vi "LinearSystemLoop_ClampInput.vi"(9 "UnclampedU":T1, 11 "input inear System Loop":T2) -> (3 "U":T1)   [LabVIEW 2019, in "Trajectory_Library.lvlib"]
doc: "Creates a new LINEAR SYSTEM data cluster with the specified values. \n\n\nInputs: \n - XXX -- XXX.\n\nOutputs:\n - XXX -- XXX."
uses:
  Trajectory_Library.lvlib
  <vilib>/Analysis/Matrix/Datatypes/RealMatrix.ctl
  LINEAR_SYSTEM_LOOP.ctl
  LINEAR_QUADRATIC_REGULATOR.ctl
  LINEAR_PLANT_INV_FF.ctl
  KALMAN_FILTER.ctl
  LINEAR_SYSTEM.ctl
  <vilib>/Analysis/Matrix/NI_Matrix.lvlib
panel:
  # "<States,1>"
  # "<FUTURE --- CLAMP TYPE -- For now\nuse Normalize>"
  # "Steady State Gain  \n<States,Outputs>"
  # "State Estimate <Statess,1>"
  # "<States,States>"
  # "<States,Inputs>"
  # "<Outputs,States>"
  # "<Outputs,Inputs>"
  # "<States,1>"
  # "<Inputs,1>"
  # "<States,Inputs>"
  # "<States,States>"
  # "Ref State <States,1>"
  # "Comp and capped \noutput <Inputs,1>"
  # "Controller gain\n<Inputs,States>"
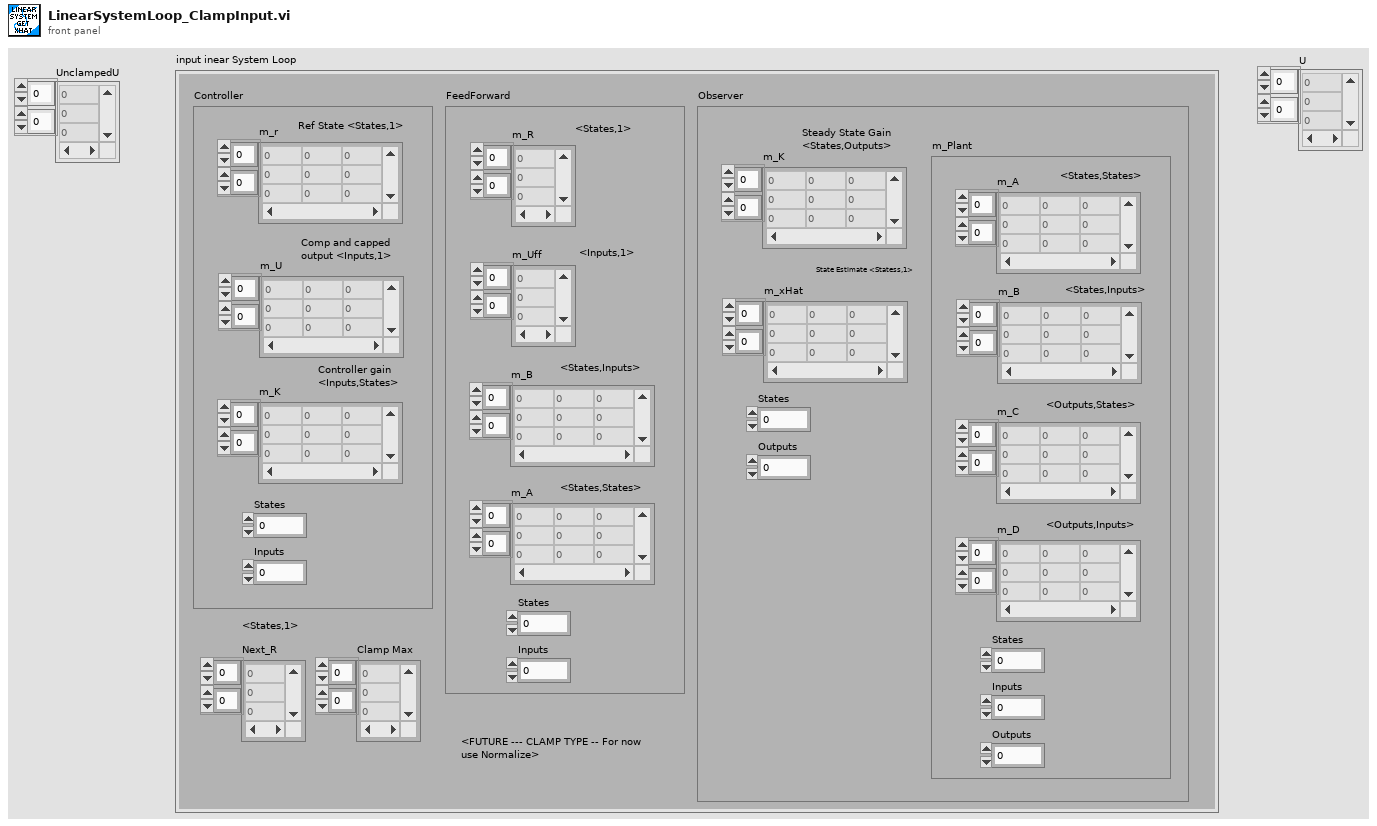
[diagram p1: front panel]
types:
  T1 = typedef "NI_Matrix.lvlib/RealMatrix.ctl" = dbl[][]
  T2 = typedef "Trajectory_Library.lvlib/LINEAR_SYSTEM_LOOP.ctl" = cluster{"Controller":T3, "FeedForward":T4, "Observer":T5, "Next_R":T1, "Clamp Max":T1}
  T3 = typedef "Trajectory_Library.lvlib/LINEAR_QUADRATIC_REGULATOR.ctl" = cluster{"m_r":T1, "m_U":T1, "m_K":T1, "States":i32, "Inputs":i32}
  T4 = typedef "Trajectory_Library.lvlib/LINEAR_PLANT_INV_FF.ctl" = cluster{"m_R":T1, "m_Uff":T1, "m_B":T1, "m_A":T1, "States":i32, "Inputs":i32}
  T5 = typedef "Trajectory_Library.lvlib/KALMAN_FILTER.ctl" = cluster{"m_K":T1, "m_xHat":T1, "States":i32, "Outputs":i32, "m_Plant":T6}
  T6 = typedef "Trajectory_Library.lvlib/LINEAR_SYSTEM.ctl" = cluster{"m_A":T1, "m_B":T1, "m_C":T1, "m_D":T1, "States":i32, "Inputs":i32, "Outputs":i32}
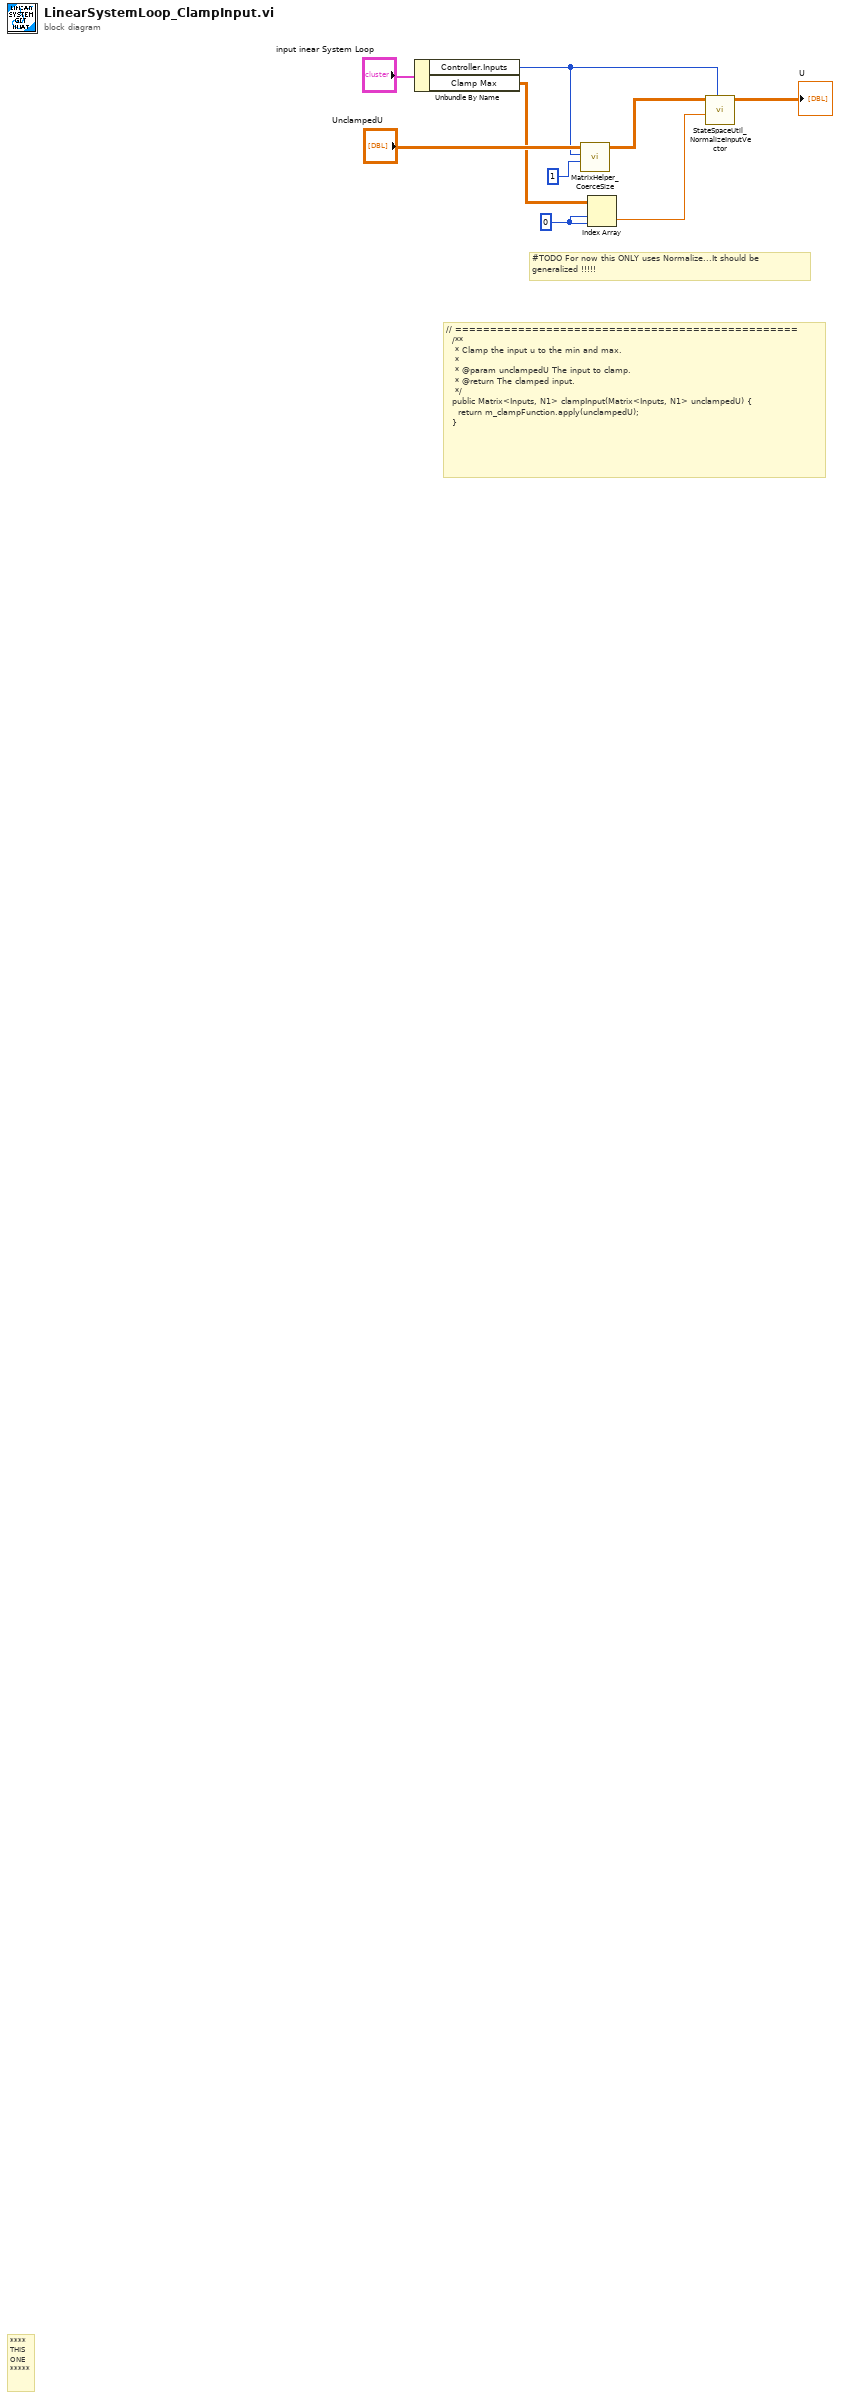
[diagram p0: block diagram]
diagram:
  w2 = 0 ("index (row)")
  # "#TODO For now this ONLY uses Normalize...It should be\ngeneralized !!!!!"
  # "// =================================================\n  /**\n   * Clamp the input u to the min and max.\n   *\n   * @param unclampedU The input to clamp.\n   * @return The clamped input.\n   */\n  public Matrix<Inputs, N1> clampInput(Matrix<Inputs, N1> unclampedU) {\n    return m_clampFunction.apply(unclampedU);\n  }"
  # "****\nTHIS\nONE\n*****"
  n1 = Unbundle By Name("input inear System Loop") -> ("Controller.Inputs"=w5:i32, "Clamp Max"=w3:T1)
  n2 = call "MatrixHelper_CoerceSize.vi"("Columns"=1, "Rows"=w5, "input matrix"="UnclampedU") -> ("output matrix"=w6:T1)  [unwired: 8 in]
  n3 = Index Array(array=w3, index (row)=w2, index (col)=w2) -> (element=w1:dbl)
  n4 = call "StateSpaceUtil_NormalizeInputVector.vi"("J"=w5, "Max_Magnitude"=w1, "U"=w6) -> ("NormalizedU"=→"U":T1)  [unwired: 8 in]
